vi "Variable@SUnion__Parameter.vi"(1 "ParamterIn":string) -> (0 "ParamterOut":string)   [LabVIEW 2020]
panel:
  in  "Var2":string(combo)
  in  "Section":string(combo)
  in  "Var1":string(combo)
  in  "ParameterName":string(combo)
  in  "Confirm":bool
  # "Variable@SUnion $Variable,$Var1,$Var2(,$Section)"
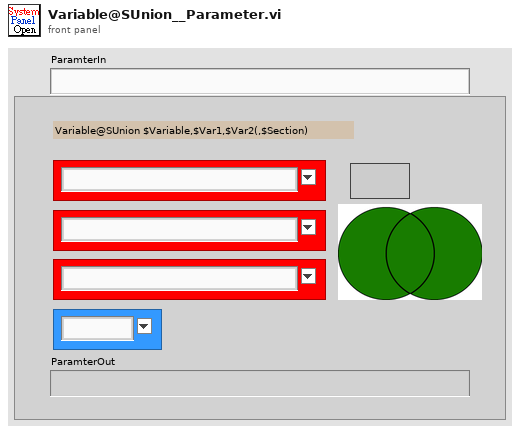
[diagram p1: front panel]
types:
  T1 = enum16{"Get", "Init", "Set", "Delete", "GetElement", "Inc", "Dec", "ReName"}
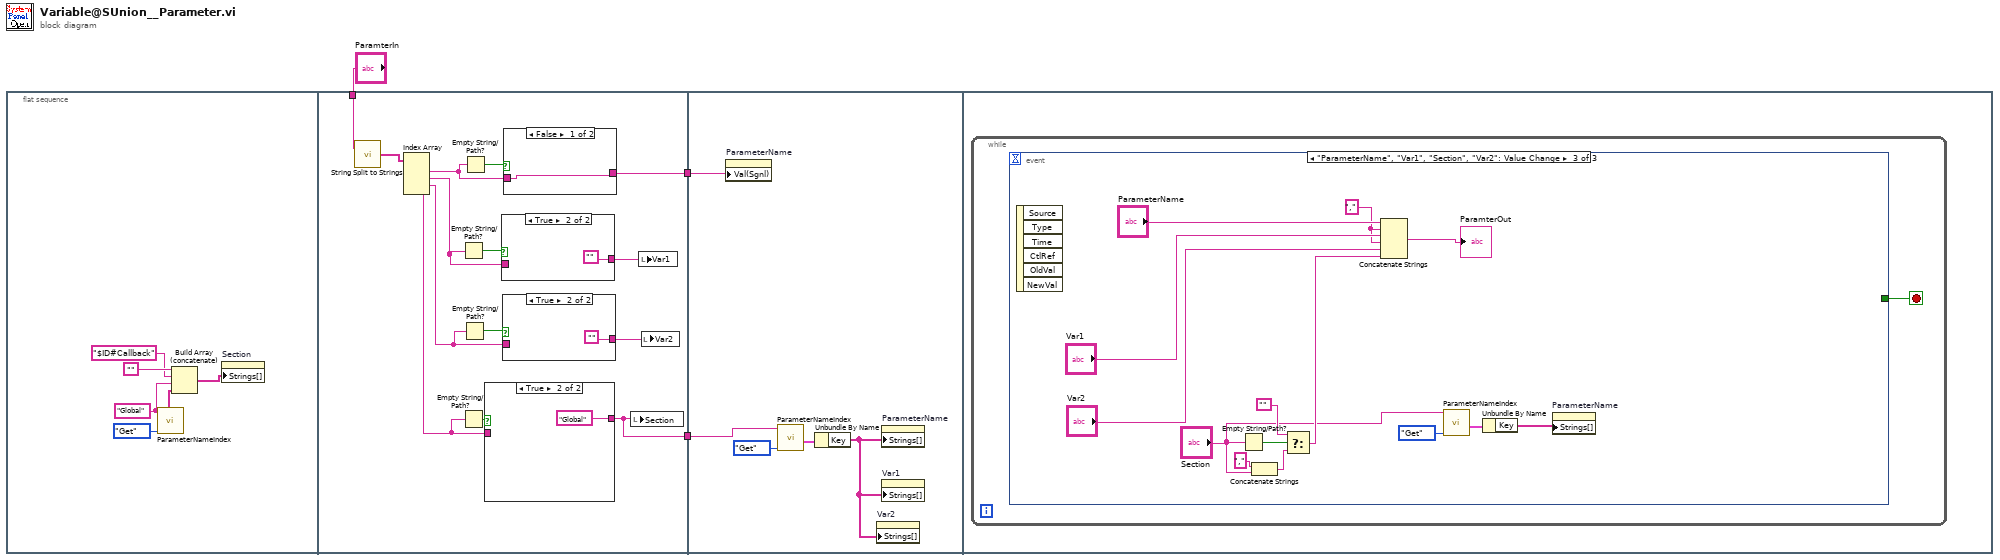
[diagram p0: block diagram]
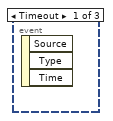
[diagram p6: hidden frame]
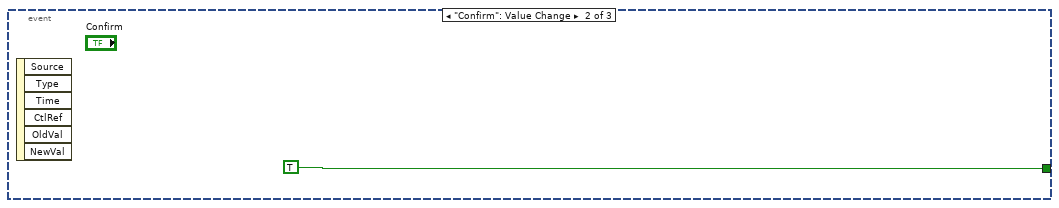
[diagram p7: hidden frame]
diagram:
  n1 = flat-sequence {
    tunnel: "ParamterIn" -> [w19]
    tunnel: [w21] -> w2
    tunnel: [w10] -> w1
    tunnel: w2 -> [w36]
    tunnel: w1 -> [w32]
    frame #0 {
      w6 = "Global" ("VariableSection")
      n2 = call "ParameterNameIndex.vi"("OP"=T1."Get", "VariableSection"=w6) -> ("SectionList"=w7:string[])  [unwired: 3 in, 6 out]
      n3 = Build Array (concatenate)("", "$ID#Callback" ("VariableSection"), w6, w7) -> (w5:string[])
      n4 = property on="Section" class="CmbBox"("Strings[]"=w5) -> ()  [unwired: 2 in, 2 out]
    }
    frame #1 {
      n5 = call "String Split to Strings.vi"("String"=w19) -> ("Array"=w18:string[])  [unwired: 1 in]
      n6 = Index Array(array=w18) -> (element #1=w17:string, element #2=w16:string, element #3=w11:string, element #4=w14:string)  [unwired: 4 in]
      n7 = Empty String/Path?(string/path=w16) -> (empty?=w22:bool)
      n8 = Empty String/Path?(string/path=w14) -> (empty?=w15:bool)
      n9 = Empty String/Path?(string/path=w11) -> (empty?=w13:bool)
      n10 = Empty String/Path?(string/path=w17) -> (empty?=w23:bool)
      n11 = case shown="True" w15 {
        tunnel: w14 -> [w26 _]
        tunnel: [w26 "Global"] -> w10
        frame False {
        }
        frame True {
        }
      }
      n12 = case shown="True" w22 {
        tunnel: w16 -> [w28 _]
        tunnel: [w28 ""] -> w20
        frame False {
        }
        frame True {
        }
      }
      n13 = case shown="True" w13 {
        tunnel: w11 -> [w24 _]
        tunnel: [w24 ""] -> w12
        frame False {
        }
        frame True {
        }
      }
      n14 = case shown="False" w23 {
        tunnel: w17 -> [w30 w31]
        tunnel: [w30 w31] -> w21
        frame False {
        }
        frame True {
        }
      }
      n15 = local write "Section"(w10) -> ()
      n16 = local write "Var1"(w20) -> ()
      n17 = local write "Var2"(w12) -> ()
    }
    frame #2 {
      n18 = property on="ParameterName" class="CmbBox"("Val(Sgnl)"=w36) -> ()  [unwired: 2 in, 2 out]
      n19 = call "ParameterNameIndex.vi"("OP"=T1."Get", "VariableSection"=w32) -> ("GlobalKeyValue"=w34:cluster{"Key":string[], "Value":string[]})  [unwired: 3 in, 6 out]
      n20 = Unbundle By Name(w34) -> ("Key"=w35:string[])
      n21 = property on="Var2" class="CmbBox"("Strings[]"=w35) -> ()  [unwired: 2 in, 2 out]
      n22 = property on="ParameterName" class="CmbBox"("Strings[]"=w35) -> ()  [unwired: 2 in, 2 out]
      n23 = property on="Var1" class="CmbBox"("Strings[]"=w35) -> ()  [unwired: 2 in, 2 out]
    }
    frame #3 {
      n24 = while {
        stop <- w37 stop-if-true
        n25 = event shown="[2] \"ParameterName\", \"Var1\", \"Section\", \"Var2\": Value Change" {
          selector: _ -> [_ _ _]
          dyn-events: _ -> [_ _ _]
          timeout: _ -> [_ _ _]
          tunnel: [_ TRUE _] -> w37
          event Timeout {
            n26 = event-data() -> ()  [unwired: 1 in, 3 out]
          }
          event "Confirm": Value Change {
            n27 = event-data() -> ()  [unwired: 1 in, 6 out]
          }
          event "ParameterName", "Var1", "Section", "Var2": Value Change {
            w44 = "," ("string")
            n28 = event-data() -> ()  [unwired: 1 in, 6 out]
            n29 = Empty String/Path?(string/path="Section") -> (empty?=w48:bool)
            n30 = Concatenate Strings("," ("string"), "Section") -> (w49:string)
            n31 = Select(t="", s=w48, f=w49) -> (s? t:f=w42:string)
            n32 = Concatenate Strings("ParameterName", w44, "Var1", w44, "Var2", w42) -> (→"ParamterOut":string)
            n33 = call "ParameterNameIndex.vi"("OP"=T1."Get", "VariableSection"="Section") -> ("GlobalKeyValue"=w40:cluster{"Key":string[], "Value":string[]})  [unwired: 3 in, 6 out]
            n34 = Unbundle By Name(w40) -> ("Key"=w47:string[])
            n35 = property on="ParameterName" class="CmbBox"("Strings[]"=w47) -> ()  [unwired: 2 in, 2 out]
          }
        }
      }
    }
  }
